vi "Reporting Interval.vi"(7 "Reporting Interval (s)":dbl=10.0 caption="Time Target (s)", 11 "Report Enable":T1) -> (3 "Report Data":T1)   [LabVIEW 2014]
uses:
  Controls/Enable Voice Reporting.ctl
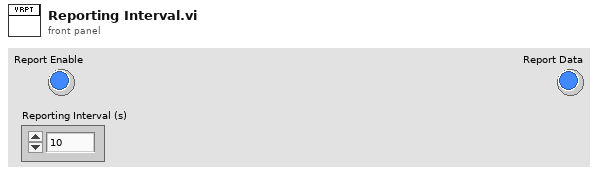
[diagram p1: front panel]
types:
  T1 = typedef "Enable Voice Reporting.ctl" = bool
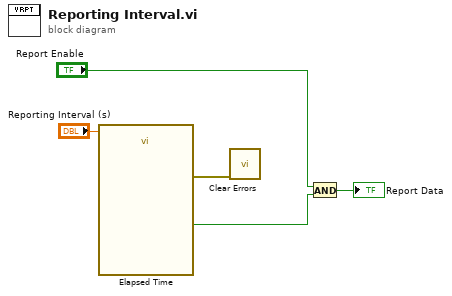
[diagram p0: block diagram]
diagram:
  n1 = call "Elapsed Time"("Time Target (s)"="Reporting Interval (s)") -> ("Time has Elapsed"=w4:bool, "error out"=w1:errorcluster)  [unwired: 11 in, 6 out]
  n2 = call <vilib>:"Clear Errors.vi"("error in (no error)"=w1) -> ()  [unwired: 5 in, 2 out]
  n3 = And(x="Report Enable", y=w4) -> (x .and. y?=→"Report Data":T1)
